vi "testing.vi"() -> ()   [LabVIEW 2017, in "LabVIEW NPOI.lvlib" / "MS-Excel.lvclass"]
uses:
  MS-Excel.lvclass
  C:/Users/Neo/Desktop/Dev_Tools_BR/LabVIEW_NPOI/src/LabVIEW NPOI/Document/Document.lvclass
  Styles/Style--cluster.ctl
  Styles/Font--cluster.ctl
  Styles/Underline--ring.ctl
  Styles/Alignment--ring.ctl
  Document/Read Table As String.vi
  Append 1D Column Timestamp.vi
  Append 1D Column Boolean.vi
  Document/Document.lvclass
  Styles/Styles.lvlib
panel:
  out "double precision float":dbl
  out "Table":string[][](array[string])
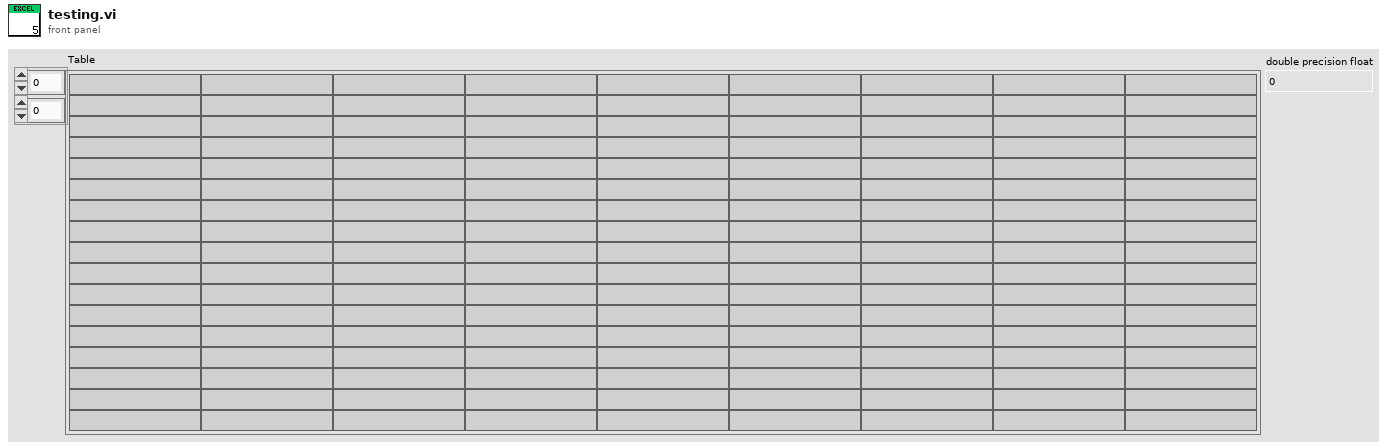
[diagram p1: front panel]
types:
  T1 = typedef "Styles.lvlib/Style--cluster.ctl" = cluster{"Name":string, "Font":T2}
  T2 = typedef "Styles.lvlib/Font--cluster.ctl" = cluster{"Name":string, "Size":i32, "Bold":bool, "Italic":bool, "Underline":T3, "Strike":bool, "Color":u32, "Alignment":T4}
  T3 = typedef "Styles.lvlib/Underline--ring.ctl" = i32
  T4 = typedef "Styles.lvlib/Alignment--ring.ctl" = i32
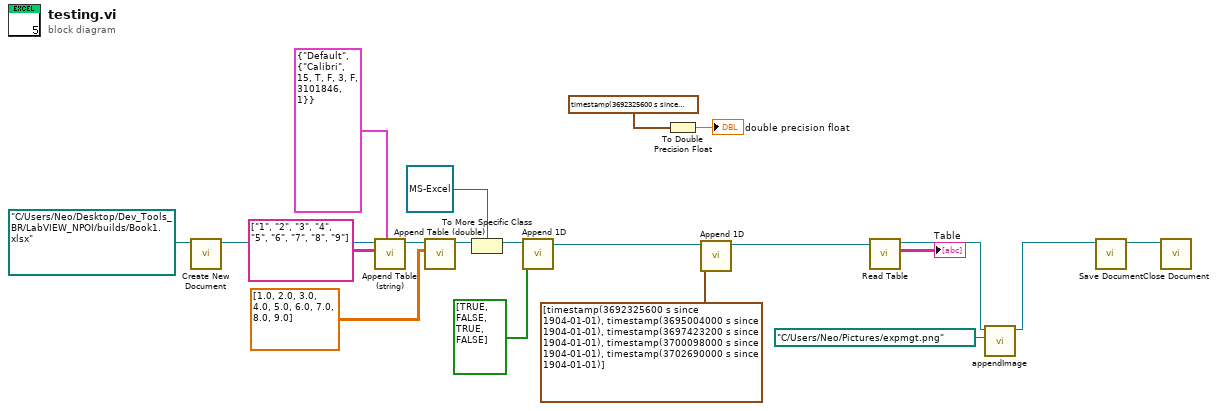
[diagram p0: block diagram]
diagram:
  n1 = call "Create New Document.vi"("File Path"=path "C:/Users/Neo/Desktop/Dev_Tools_BR/LabVIEW_NPOI/builds/Book1.xlsx") -> ("Document out"=w20:refnum<class "Document.lvclass">)  [unwired: 9 in, 1 out]
  n2 = call "Append Table (string).vi"("Style"=T1 {"Name"="Default", "Font"={"Name"="Calibri", "Size"=15, "Bold"=TRUE, "Italic"=FALSE, "Underline"=3, "Strike"=FALSE, "Color"=3101846, "Alignment"=1}}, "Table"=string[][] [["1", "2", "3"], ["4", "5", "6"], ["7", "8", "9"]], "Document in"=w20) -> ("Document out"=w15:refnum<class "Document.lvclass">)  [unwired: 7 in, 1 out]
  n3 = call "Append Table (double).vi"("Table"=dbl[][] [[1.0, 2.0, 3.0], [4.0, 5.0, 6.0], [7.0, 8.0, 9.0]], "Document in"=w15) -> ("Document out"=w12:refnum<class "Document.lvclass">)  [unwired: 8 in, 1 out]
  n4 = To More Specific Class(target class=refnum<class "MS-Excel.lvclass"> refnum ("LabVIEW NPOI.lvlib:MS-Excel.lvclass"), reference=w12) -> (specific class reference=w5:refnum<class "MS-Excel.lvclass">)  [unwired: 1 in, 1 out]
  n5 = call-poly "Append 1D.vi"("Value"=bool[] [TRUE, FALSE, TRUE, FALSE], "MS-Excel in"=w5) -> ("MS-Excel out"=w10:refnum<class "MS-Excel.lvclass">)  [unwired: 8 in, 1 out]
  n6 = To Double Precision Float(number=timestamp(3692325600 s since 1904-01-01) ("Time Stamp")) -> (double precision float=→"double precision float":dbl)
  n7 = call-poly "Append 1D.vi"("Value"=timestamp[] [timestamp(3692325600 s since 1904-01-01), timestamp(3695004000 s since 1904-01-01), timestamp(3697423200 s since 1904-01-01), timestamp(3700098000 s since 1904-01-01), timestamp(3702690000 s since 1904-01-01)], "MS-Excel in"=w10) -> ("MS-Excel out"=w18:refnum<class "MS-Excel.lvclass">)  [unwired: 8 in, 1 out]
  n8 = call-poly "Read Table.vi"("Document in"=w18) -> ("Table As String"=→"Table":string[][], "Document out"=w3:refnum<class "MS-Excel.lvclass">)  [unwired: 8 in, 1 out]
  n9 = call-dynamic "appendImage.vi"("Image Path"=path "C:/Users/Neo/Pictures/expmgt.png" ("file (use dialog)"), "MS-Excel in"=w3) -> ("MS-Excel out"=w2:refnum<class "MS-Excel.lvclass">)  [unwired: 8 in, 1 out]
  n10 = call "Save Document.vi"("Document in"=w2) -> ("Document out"=w17:refnum<class "MS-Excel.lvclass">)  [unwired: 9 in, 1 out]
  n11 = call "Close Document.vi"("Document in"=w17) -> ()  [unwired: 10 in, 1 out]
